vi "GetArray.vi"(8 "error in (no error)":errorcluster, 10 "size":i32, 11 "MsgPackDeserializer in":refnum<class "MsgPackDeserializer.lvclass">) -> (0 "error out":errorcluster, 2 "Variant":variant, 3 "MsgPackDeserializer out":refnum<class "MsgPackDeserializer.lvclass">)   [LabVIEW 2015, in "MsgPackDeserializer.lvclass"]
uses:
  MsgPackDeserializer.lvclass
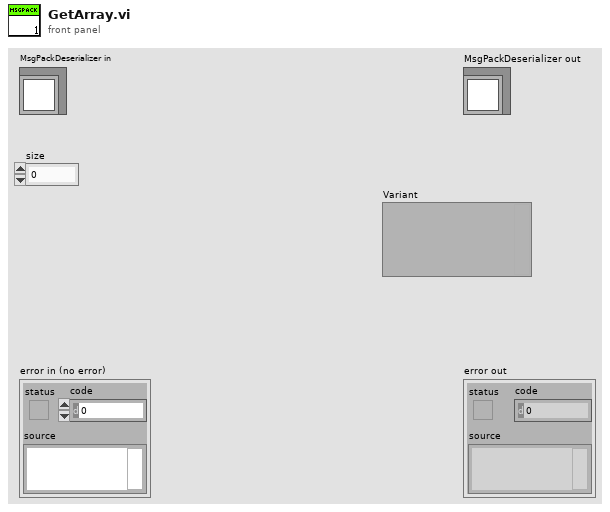
[diagram p1: front panel]
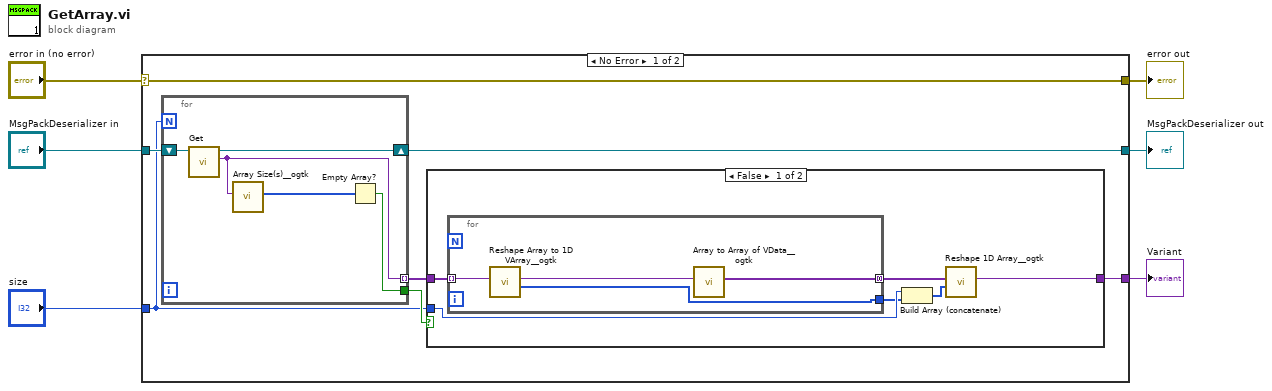
[diagram p0: block diagram]
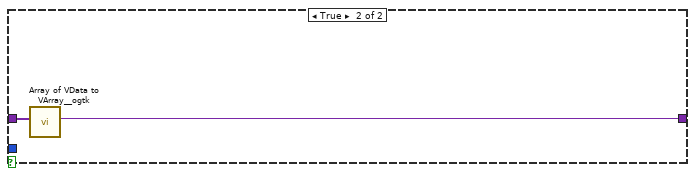
[diagram p2: hidden frame]
diagram:
  n1 = case shown="No Error" "error in (no error)" {
    selector: "error in (no error)" -> [w13 w32]
    tunnel: [w13 w32] -> w5
    tunnel: [w11 w31] -> w3
    tunnel: "MsgPackDeserializer in" -> [w12 w31]
    tunnel: "size" -> [w7 _]
    tunnel: [w8 _] -> w1
    frame No Error {
      n2 = for {
        N: w7 -> [_]
        shift-right: [w29] -> w11
        shift-left: w12 -> [w30]
        tunnel: [w27] -> w9 mode=indexing
        tunnel: [w26] -> w10
        n3 = call "Get.vi"("MsgPackDeserializer in"=w30) -> ("Variant"=w27:variant, "MsgPackDeserializer out"=w29:refnum<class "MsgPackDeserializer.lvclass">)  [unwired: 8 in, 1 out]
        n4 = call <userlib>:"Array Size(s)__ogtk.vi"("Array"=w27) -> ("Size(s)"=w28:u32[])  [unwired: 8 in, 2 out]
        n5 = Empty Array?(array=w28) -> (empty?=w26:bool)
      }
      n6 = case shown="False" w10 {
        tunnel: w9 -> [w18 w25]
        tunnel: [w14 w24] -> w8
        tunnel: w7 -> [w17 _]
        frame False {
          n7 = for {
            tunnel: [w23] -> w19 mode=concatenating
            tunnel: w18 -> [w22] mode=indexing
            tunnel: [w20] -> w16
            n8 = call <userlib>:"Reshape Array to 1D VArray__ogtk.vi"("MultiD Array"=w22) -> ("Size(s)"=w20:u32[], "1D VArray"=w21:variant)  [unwired: 8 in, 1 out]
            n9 = call <userlib>:"Array to Array of VData__ogtk.vi"("MultiD Array"=w21) -> ("1D Array of Variants"=w23:variant[])  [unwired: 9 in, 1 out]
          }
          n10 = Build Array (concatenate)(w17, w16) -> (w15:u32[])
          n11 = call <userlib>:"Reshape 1D Array__ogtk.vi"("Size(s)"=w15, "1D Array"=w19) -> ("Reshaped VArray"=w14:variant)  [unwired: 8 in, 1 out]
        }
        frame True {
          n12 = call <userlib>:"Array of VData to VArray__ogtk.vi"("1D Array of VData"=w25) -> ("VArray"=w24:variant)  [unwired: 9 in, 1 out]
        }
      }
    }
    frame Error {
    }
  }
  "error out" <- w5
  "MsgPackDeserializer out" <- w3
  "Variant" <- w1
